vi "Reset Graph.vi"(3 "error in (no error)":errorcluster, 4 "Graph Boundaries":T1, 5 "Graph Reference":refnum<vi>) -> (0 "error out":errorcluster)   [LabVIEW 2013]
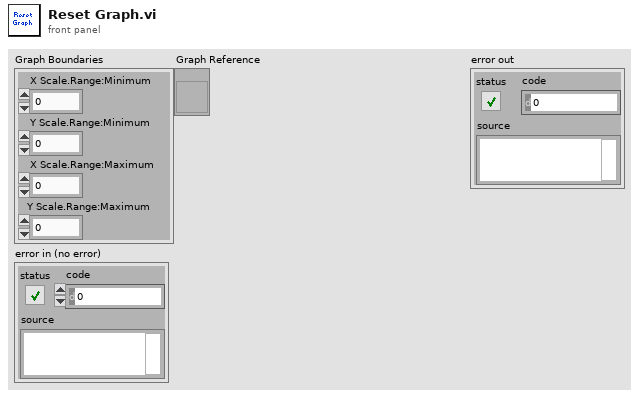
[diagram p1: front panel]
types:
  T1 = cluster{"X Scale.Range:Minimum":dbl, "Y Scale.Range:Minimum":dbl, "X Scale.Range:Maximum":dbl, "Y Scale.Range:Maximum":dbl}
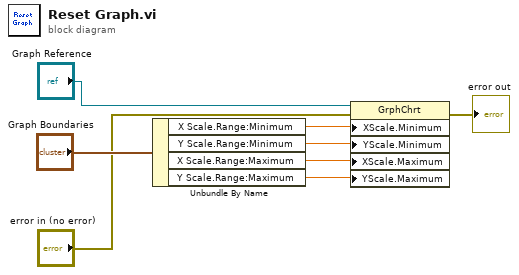
[diagram p0: block diagram]
diagram:
  n1 = Unbundle By Name("Graph Boundaries") -> ("X Scale.Range:Minimum"=w8:dbl, "Y Scale.Range:Minimum"=w7:dbl, "X Scale.Range:Maximum"=w6:dbl, "Y Scale.Range:Maximum"=w5:dbl)
  n2 = property on="Property Node" class="GrphChrt"(reference="Graph Reference", error in="error in (no error)", "XScale.Minimum"=w8, "YScale.Minimum"=w7, "XScale.Maximum"=w6, "YScale.Maximum"=w5) -> (error out=→"error out":errorcluster)  [unwired: 1 out]
